vi "Configure Generator Digital Gain.vi"(8 "error in (no error)":errorcluster, 9 "Digital Gain (0.0)":dbl format="%^.3e", 10 "Instance (1)":i32=1, 11 "VISA resource name":refnum<visa-resource-name>) -> (0 "error out":errorcluster, 3 "VISA resource name out":refnum<visa-resource-name>)   [LabVIEW 2015, in "Rohde&Schwarz CMXP GPRF.lvlib"]
doc: "Defines or the digital gain of the constant-frequency RF generator.\n\nAttribute:\nRSCMXPGPRF_ATTR_GENERATOR_DIGITAL_GAIN\n\nRemote-control command:\nSOURce:GPRF:GEN<i>:RFSettings:DGAin"
uses:
  <instrlib>/Rohde&Schwarz CMXP GPRF/Rohde&Schwarz CMXP GPRF.lvlib
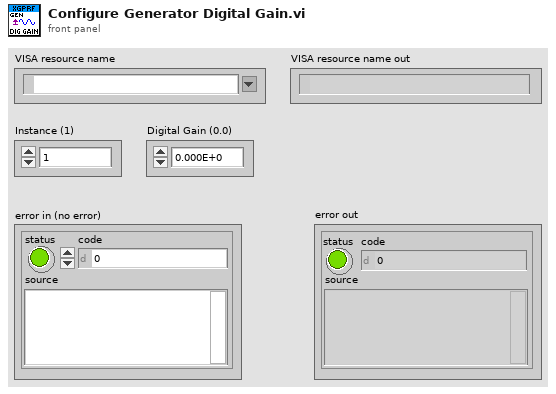
[diagram p1: front panel]
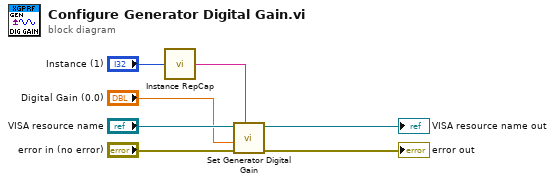
[diagram p0: block diagram]
diagram:
  n1 = call <instrlib>:"Instance RepCap.vi"("instance  in"="Instance (1)") -> ("instance out"=w6:string)
  n2 = call "Set Generator Digital Gain"("Repeated Capabilities"=w6, "error in (no error)"="error in (no error)", "Generator Digital Gain (0.0)"="Digital Gain (0.0)", "instrument handle"="VISA resource name") -> ("error out"=→"error out":errorcluster, "instrument handle out"=→"VISA resource name out":refnum<visa-resource-name>)  [unwired: 6 in]
